vi "Image Paths--constant.vi"() -> (3 "Array":path[](array[path]))   [LabVIEW 2024, in "UIs Handler.lvlib"]
uses:
  UIs Handler.lvlib
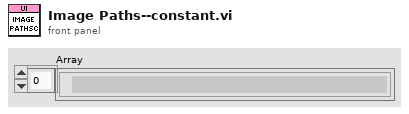
[diagram p1: front panel]
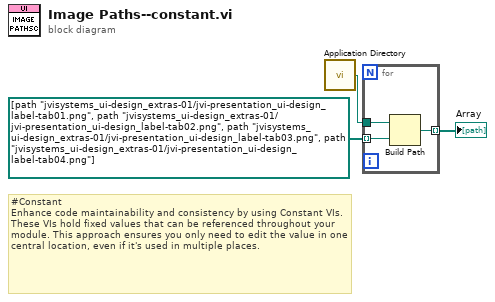
[diagram p0: block diagram]
diagram:
  # "#Constant\nEnhance code maintainability and consistency by using Constant VIs. These VIs hold fixed values that can be referenced throughout your module. This approach ensures you only need to edit the value in one central location, even if it's used in multiple places."
  n1 = call <vilib>:"Application Directory.vi"() -> ("Application Directory"=w3:path)
  n2 = for {
    tunnel: w3 -> [w6]
    tunnel: path[] [path "jvisystems_ui-design_extras-01/jvi-presentation_ui-design_label-tab01.png", path "jvisystems_ui-design_extras-01/jvi-presentation_ui-design_label-tab02.png", path "jvisystems_ui-design_extras-01/jvi-presentation_ui-design_label-tab03.png", path "jvisystems_ui-design_extras-01/jvi-presentation_ui-design_label-tab04.png"] ("Array") -> [w5] mode=indexing
    tunnel: [w4] -> w1 mode=indexing
    n3 = Build Path(base path=w6, name or relative path=w5) -> (appended path=w4:path)
  }
  "Array" <- w1
